vi "Updated Command Status.vi"(8 "error in (no error)":errorcluster, 10 "Command Status":T1, 11 "System Actor in":refnum<class "System Actor.lvclass">) -> (0 "error out":errorcluster, 3 "System Actor out":refnum<class "System Actor.lvclass">)   [LabVIEW 2013, in "Robot Actors.lvlib" / "System Actor.lvlib" / "System Actor.lvclass"]
uses:
  System Actor.lvclass
  Command/Command Class/Command Status.ctl
  Command/Command Class/Command States.ctl
  Command/Command Class/Command.lvclass
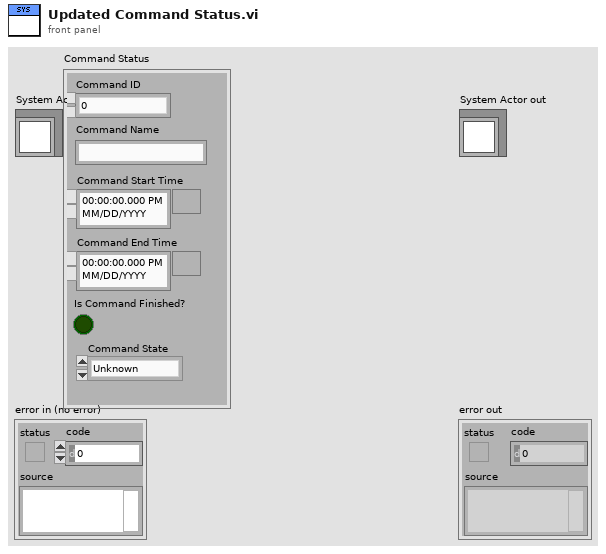
[diagram p1: front panel]
types:
  T1 = typedef "Robot Actors.lvlib/Command.lvlib/Command.lvclass/Command Status.ctl" = cluster{"Command Name":string, "Command Start Time":timestamp, "Command End Time":timestamp, "Is Command Finished?":bool, "Command ID":dbl, "Command State":T2}
  T2 = typedef "Robot Actors.lvlib/Command.lvlib/Command.lvclass/Command States.ctl" = enum16{"Unknown", "Started", "Stopped", "Finished"}
  T3 = typedef "Robot Actors.lvlib/System Actor.lvlib/System Actor.lvclass/System Status.ctl" = cluster{"Instance Name":string, "Command Status":T1, "System Start Time":timestamp, "Next Command ID":dbl}
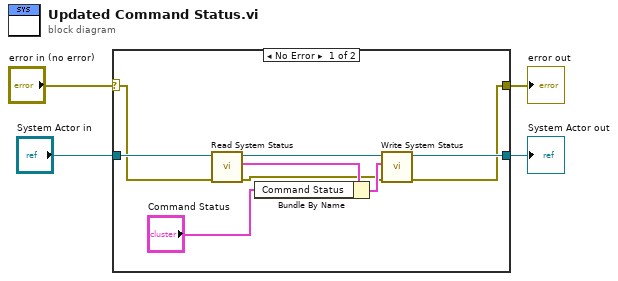
[diagram p0: block diagram]
diagram:
  n1 = case shown="No Error" "error in (no error)" {
    selector: "error in (no error)" -> [w7 w15]
    tunnel: [w5 w15] -> w3
    tunnel: [w8 w14] -> w1
    tunnel: "System Actor in" -> [w9 w14]
    frame No Error {
      n2 = call-dynamic "Read System Status.vi"("error in (no error)"=w7, "System Actor in"=w9) -> ("error out"=w6:errorcluster, "System Status"=w12:T3, "System Actor out"=w13:refnum<class "System Actor.lvclass">)  [unwired: 7 in]
      n3 = Bundle By Name(cluster=w12, "Command Status"="Command Status") -> (w11:T3)
      n4 = call-dynamic "Write System Status.vi"("error in (no error)"=w6, "System Status"=w11, "System Actor in"=w13) -> ("error out"=w5:errorcluster, "System Actor out"=w8:refnum<class "System Actor.lvclass">)  [unwired: 7 in]
    }
    frame Error {
    }
  }
  "error out" <- w3
  "System Actor out" <- w1
